vi "Read VIRef.vi"(8 "error in (no error)":errorcluster, 11 "PanelCloseMsg in":refnum<class "PanelCloseMsg.lvclass">) -> (0 "error out":errorcluster, 2 "VIRef":refnum<vi>, 3 "PanelCloseMsg out":refnum<class "PanelCloseMsg.lvclass">)   [LabVIEW 2020, in "MVA Framework.lvlib" / "ActorEvents.lvlib" / "PanelCloseMsg.lvclass"]
uses:
  PanelCloseMsg.lvclass
  PanelCloseMsg.lvclass/PanelCloseMsg.ctl
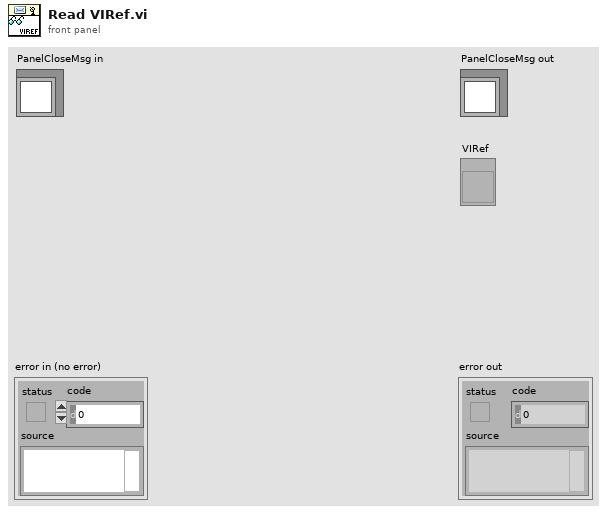
[diagram p1: front panel]
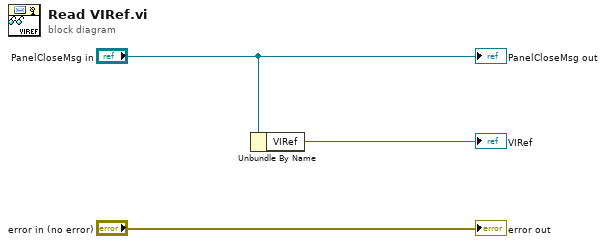
[diagram p0: block diagram]
diagram:
  n1 = Unbundle By Name("PanelCloseMsg in") -> ("VIRef"=→"VIRef":refnum<vi>)
  "error out" <- "error in (no error)"
  "PanelCloseMsg out" <- "PanelCloseMsg in"
